vi "autostage-calc-single-coordinate.vi"(0 "cycle-step":dbl, 1 "cycle-max":dbl, 2 "cycle-min":dbl, 3 "cycle-mod":i32, 4 "iterator":i32) -> (5 "current-position":dbl)   [LabVIEW 2015]
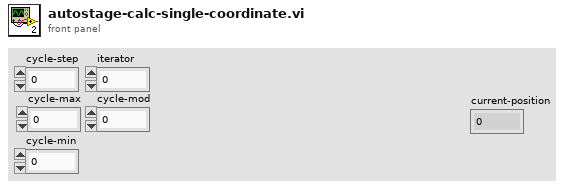
[diagram p1: front panel]
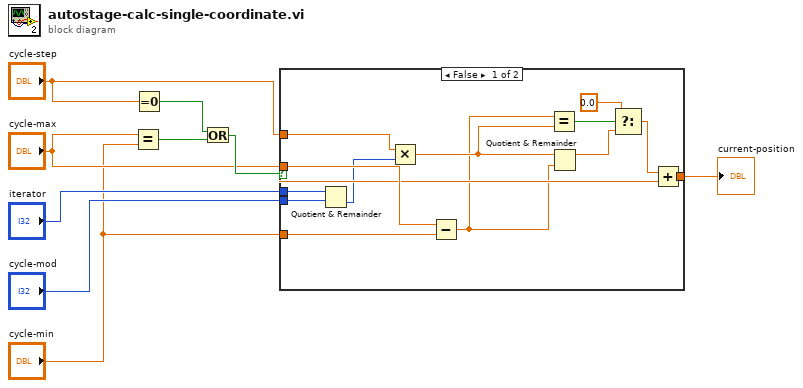
[diagram p0: block diagram]
diagram:
  n1 = Equal?(x="cycle-max", y="cycle-min") -> (x = y?=w5:bool)
  n2 = Equal To 0?(x="cycle-step") -> (x = 0?=w4:bool)
  n3 = Or(x=w4, y=w5) -> (x .or. y?=w3:bool)
  n4 = case shown="False" w3 {
    tunnel: "cycle-mod" -> [w22 _]
    tunnel: "cycle-max" -> [w21 _]
    tunnel: "cycle-min" -> [w20 w23]
    tunnel: "iterator" -> [w19 _]
    tunnel: [w18 w23] -> w6
    tunnel: "cycle-step" -> [w10 _]
    frame False {
      n5 = Quotient & Remainder(x=w19, y=w22) -> (floor(x/y)=w17:i32)  [unwired: 1 out]
      n6 = Multiply(x=w10, y=w17) -> (x*y=w15:dbl)
      n7 = Subtract(x=w21, y=w20) -> (x-y=w14:dbl)
      n8 = Equal?(x=w14, y=w15) -> (x = y?=w16:bool)
      n9 = Quotient & Remainder(x=w15, y=w14) -> (x-y*floor(x/y)=w12:dbl)  [unwired: 1 out]
      n10 = Select(t=0.0, s=w16, f=w12) -> (s? t:f=w11:dbl)
      n11 = Add(x=w11, y=w20) -> (x+y=w18:dbl)
    }
    frame True {
    }
  }
  "current-position" <- w6
